vi "Launch Test Actor.vi"(11 "RDS Root Actor in":refnum<class "RDS Root Actor.lvclass">) -> (3 "RDS Root Actor out":refnum<class "RDS Root Actor.lvclass">)   [LabVIEW 2015, in "RDS Root Actor.lvlib" / "RDS Root Actor.lvclass"]
uses:
  RDS Root Actor.lvclass
  RDS Test Child/RDS Test Child/RDS Test Child.lvclass
  RDS Parent Actor/RDS Parent Actor/RDS Parent Actor.lvclass/RDS Parent Actor.ctl
  RDS Parent Actor/RDS Parent Actor/RDS Parent Actor.lvclass
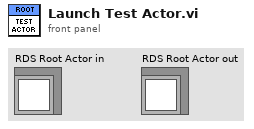
[diagram p1: front panel]
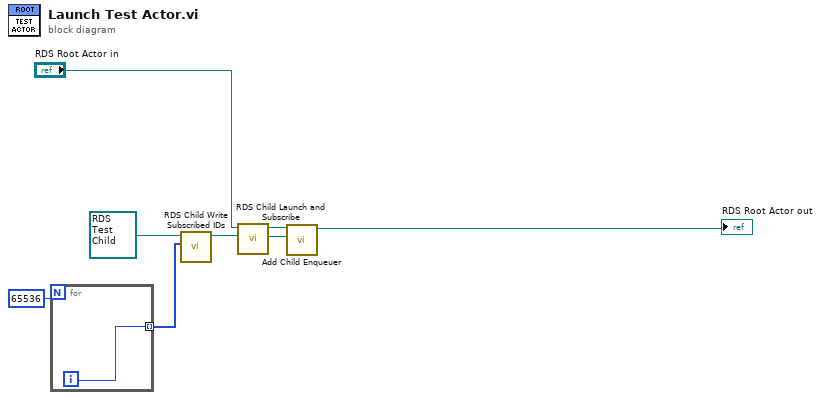
[diagram p0: block diagram]
diagram:
  n1 = for {
    N: 65536 -> [_]
    tunnel: [w9] -> w5 mode=indexing
    i -> [w9]
  }
  n2 = call "RDS Child Write Subscribed IDs.vi"("Subscribed IDs"=w5, "RDS Parent Actor in"=refnum<class "RDS Test Child.lvclass"> refnum ("RDS Test Child.lvlib:RDS Test Child.lvclass")) -> ("RDS Parent Actor out"=w4:refnum<class "RDS Test Child.lvclass">)  [unwired: 8 in, 1 out]
  n3 = call "RDS Child Launch and Subscribe.vi"("RDS Child in"=w4, "Caller Actor in"="RDS Root Actor in") -> ("Nested Actor's Enqueuer"=w7:refnum<class "Message Enqueuer.lvclass">, "Caller Actor Out"=w6:refnum<class "RDS Root Actor.lvclass">)  [unwired: 7 in, 1 out]
  n4 = call "Add Child Enqueuer.vi"("Nested Actor's Enqueuer"=w7, "RDS Root Actor in"=w6) -> ("RDS Root Actor out"=→"RDS Root Actor out":refnum<class "RDS Root Actor.lvclass">)  [unwired: 8 in, 1 out]
